vi "Host Train PID.vi"() -> ()   [LabVIEW 2018]
doc: "This example demonstrates the Traditional MeanShift algorithm to track an object in the image."
uses:
  <vilib>/userdefined/High Color/IMAQdx.ctl
  <vilib>/vision/driver/NI_Vision_Acquisition_Software.lvlib
panel:
  in  "?":T1="cam1"
  out "Control Sig":dbl(graph)
  out "Grn":bool
  out "Yel":bool
  out "Red":bool
  out "stop":bool
  out "global?":bool
  in  "Run":bool
  out "Theta":cluster{"Double":dbl, "Theta":dbl}(graph)
  out "Theta increasing?":bool
  in  "Stop":bool
  out "Image":T2(plugin-control)
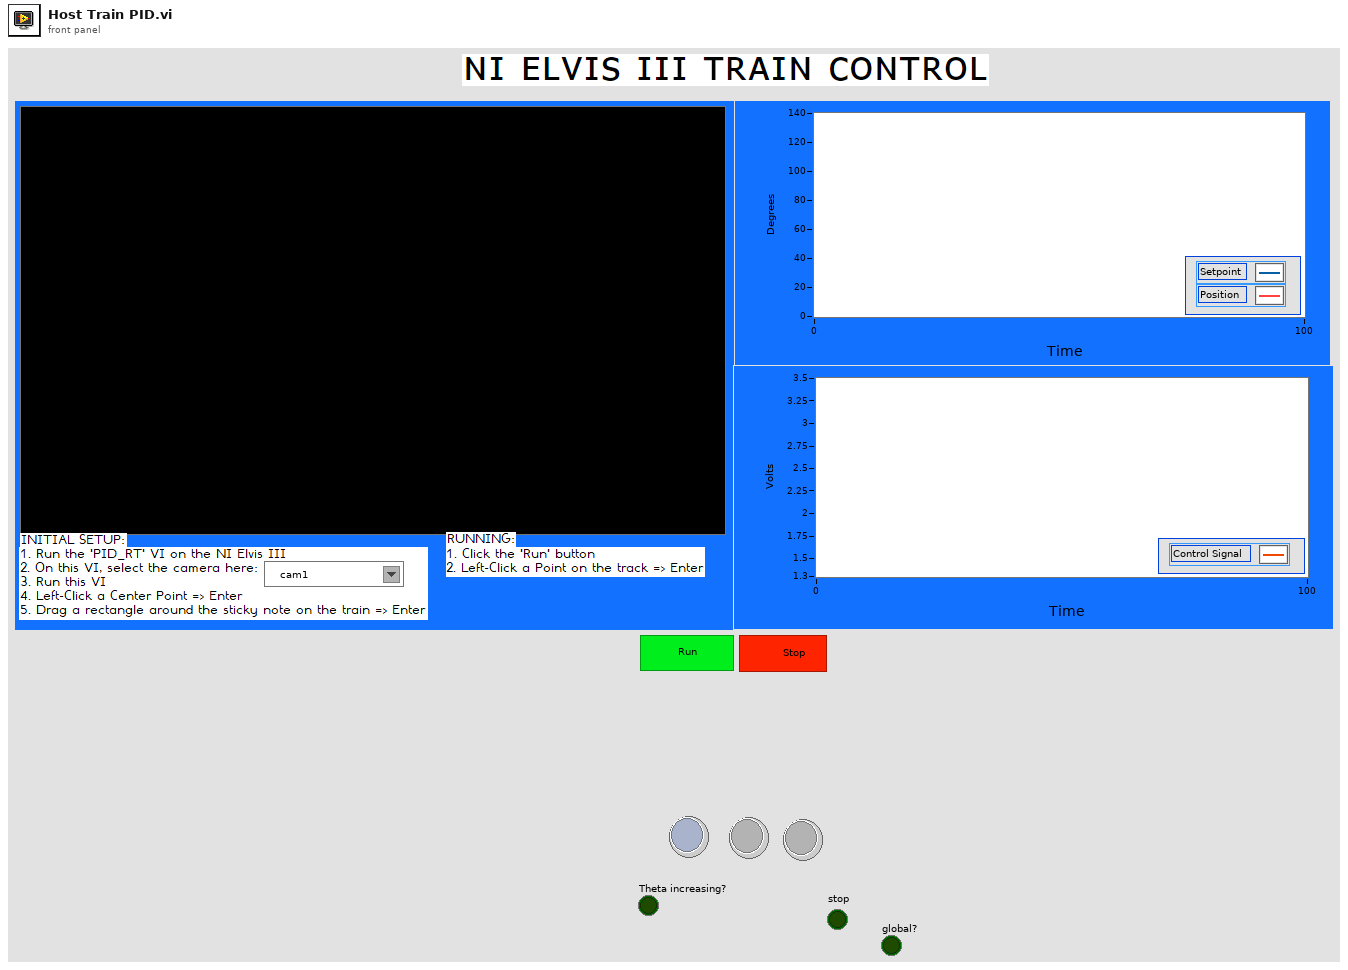
[diagram p1: front panel]
types:
  T1 = typedef "IMAQdx.ctl" = refnum<k21>
  T2 = typedef "IMAQ Image.ctl" = refnum<image>
  T3 = typedef "LVRectTypeDef.ctl" = cluster{"Left":i16, "Top":i16, "Right":i16, "Bottom":i16}
  T4 = typedef "IMAQ Object Tracking Session.ctl" = refnum<k20>
  T5 = typedef "IMAQ Point" = cluster{"X":sgl, "Y":sgl}
  T6 = cluster{"Label":string, "Score":i32, "Angle":dbl, "Location":cluster{"X":dbl, "Y":dbl}, "Bounding Box":cluster{"X":dbl, "Y":dbl}[], "Object Found?":bool}[]
  T7 = cluster{"Label":string, "Score":i32, "Angle":dbl, "Location":cluster{"X":dbl, "Y":dbl}, "Bounding Box":cluster{"X":dbl, "Y":dbl}[], "Object Found?":bool}
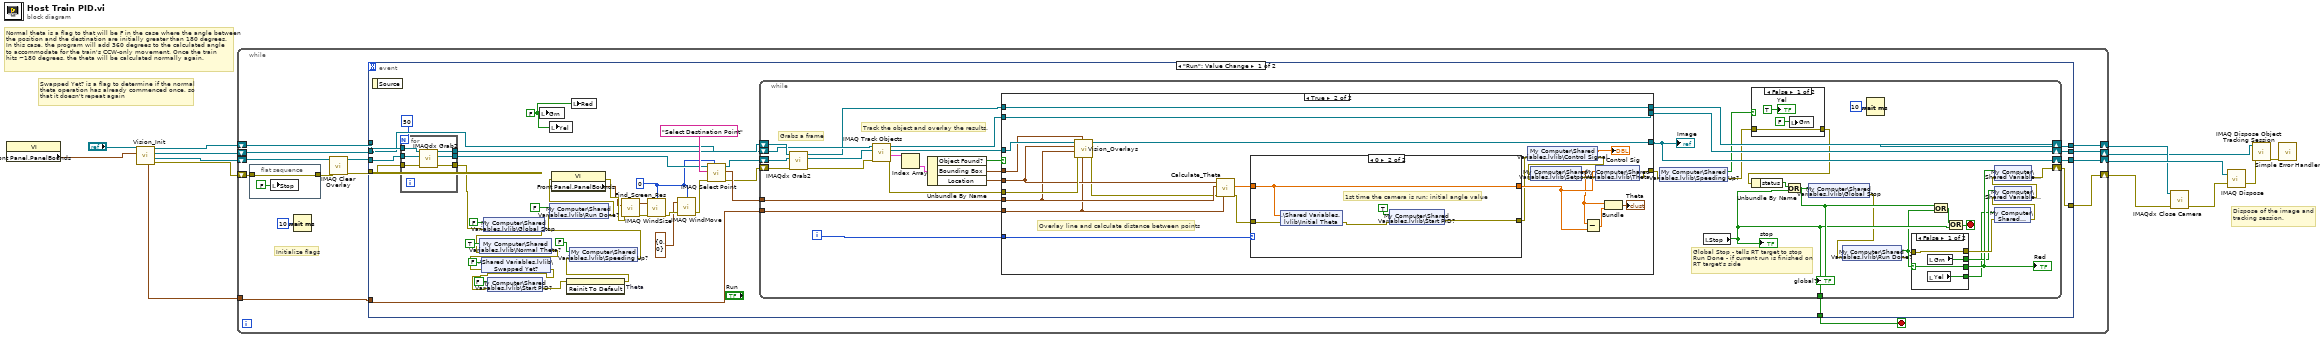
[diagram p0: block diagram]
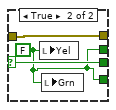
[diagram p2: hidden frame]
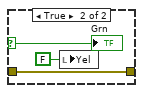
[diagram p3: hidden frame]
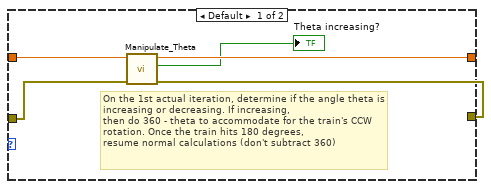
[diagram p5: hidden frame]
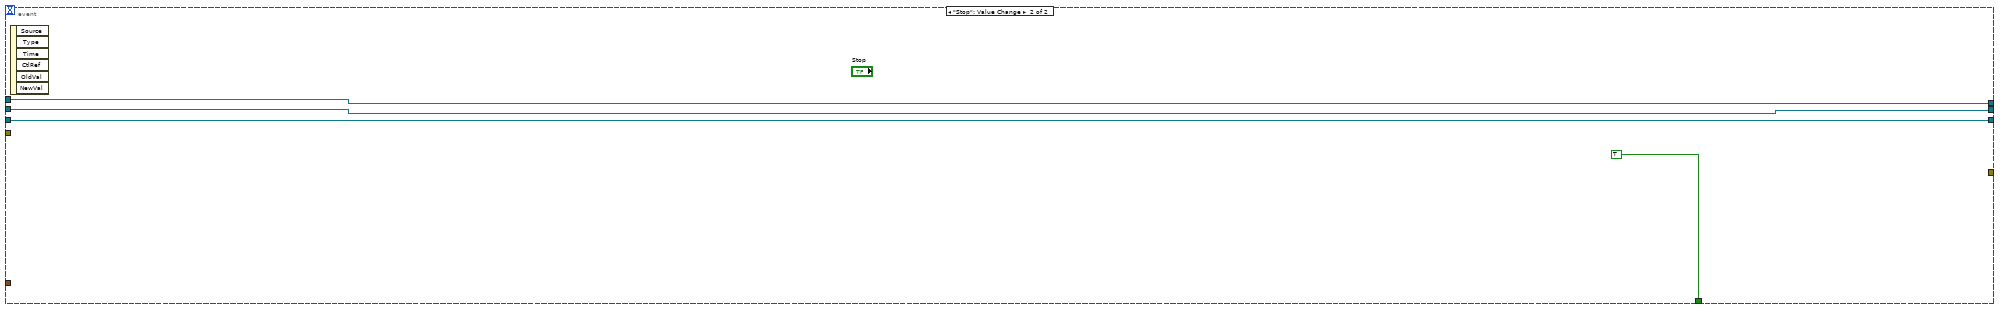
[diagram p6: hidden frame]
diagram:
  # "Swapped Yet? is a flag to determine if the normal\ntheta operation has already commenced once, so \nthat it doesn't repeat again"
  # "Normal theta is a flag to that will be F in the case where the angle between\nthe position and the destination are initially greater than 180 degrees. \nIn this case, the program will add 360 degrees to the calculated angle \nto accommodate for the train's CCW-only movement. Once the train\nhits ~180 degrees, the theta will be calculated normally again."
  # "Dispose of the image and tracking session."
  n1 = property class="VI"() -> ("Front Panel.PanelBounds"=w2:T3)  [unwired: 2 in, 2 out]
  n2 = call "Vision_Init.vi"("Front Panel.WinBounds"=w2, "Refnum in"="?") -> ("error out"=w7:errorcluster, "Image (duplicate)"=w8:T2, "Object Tracking Session Out"=w6:T4, "Refnum out"=w10:T1, "Center Point"=w5:T5)  [unwired: 5 in]
  n3 = while {
    tunnel: w5 -> [w26]
    shift-right: [w22] -> w3
    shift-left: w6 -> [w23]
    shift-right: [w28] -> w4
    shift-left: w10 -> [w24]
    shift-right: [w21] -> w9
    shift-left: w8 -> [w15]
    shift-right: [w27] -> w11
    shift-left: w7 -> [w20]
    stop <- w25 stop-if-true
    # "Initialize flags"
    n4 = flat-sequence {
      tunnel: w20 -> [w29]
      tunnel: [w29] -> w17
      frame #0 {
        n5 = local write "Stop"(FALSE ("Stop")) -> ()
      }
    }
    n6 = Wait (ms)(milliseconds to wait=u32 10) -> ()  [unwired: 1 out]
    n7 = call "IMAQ Clear Overlay"("error in (no error)"=w17, "Image"=w15) -> ("error out"=w16:errorcluster, "Image Out"=w18:T2)  [unwired: 8 in]
    n8 = event shown="[0] \"Run\": Value Change" {
      selector: _ -> [_ _]
      dyn-events: _ -> [_ _]
      timeout: _ -> [_ _]
      tunnel: w23 -> [w57 w168]
      tunnel: [w70 w169] -> w28
      tunnel: [w32 _] -> w27
      tunnel: [w69 w167] -> w21
      tunnel: w18 -> [w58 w167]
      tunnel: w26 -> [w68 _]
      tunnel: [w67 TRUE ("Stop")] -> w25
      tunnel: w24 -> [w62 w169]
      tunnel: [w63 w168] -> w22
      tunnel: w16 -> [w45 _]
      event "Run": Value Change {
        w31 = FALSE ("Grn")
        w39 = 0 ("Window Number")
        n9 = event-data() -> ()  [unwired: 1 in, 1 out]
        n10 = for {
          N: 50 -> [_]
          tunnel: w62 -> [w76]
          tunnel: [w75] -> w51
          tunnel: [w74] -> w60
          tunnel: [w73] -> w61
          tunnel: w58 -> [w72]
          tunnel: w45 -> [w71]
          n11 = call <vilib>:"IMAQdx Grab2.vi"("error in"=w71, "Image In"=w72, "Session In"=w76) -> ("error out"=w75:errorcluster, "Image Out"=w74:T2, "Session Out"=w73:T1)  [unwired: 5 in, 1 out]
        }
        n12 = shared-variable "My Computer\\Shared Variables.lvlib\\Global Stop"(FALSE ("Global Stop"), error in=w51) -> (error out=w50:errorcluster)
        n13 = shared-variable "My Computer\\Shared Variables.lvlib\\Normal Theta?"(TRUE ("Add 360?"), error in=w50) -> (error out=w49:errorcluster)
        n14 = shared-variable ".\\Shared Variables.lvlib\\Swapped Yet?"(FALSE ("Swapped Yet?"), error in=w49) -> (error out=w47:errorcluster)
        n15 = shared-variable "My Computer\\Shared Variables.lvlib\\Start PID?"(FALSE ("Start PID?"), error in=w47) -> (error out=w46:errorcluster)
        n16 = local write "Grn"(w31) -> ()
        n17 = local write "Yel"(w31) -> ()
        n18 = invoke on="Theta" class="WFChart (strict)" method="Reinit To Default"(error in=w46) -> (error out=w35:errorcluster)  [unwired: 2 in, 2 out]
        n19 = shared-variable "My Computer\\Shared Variables.lvlib\\Speeding Up?"(FALSE ("Speeding Up?"), error in=w35) -> (error out=w34:errorcluster)
        n20 = shared-variable "My Computer\\Shared Variables.lvlib\\Run Done?"(FALSE ("Run Done?"), error in=w34) -> (error out=w38:errorcluster)
        n21 = property class="VI"(error in=w38) -> (error out=w37:errorcluster, "Front Panel.PanelBounds"=w36:T3)  [unwired: 1 in, 1 out]
        n22 = local write "Red"(w31) -> ()
        n23 = call "Find_Screen_Res.vi"("error in (no error)"=w37, "Front Panel.WinBounds"=w36) -> ("error out"=w44:errorcluster, "Width & Height"=w43:cluster{"Width":i32, "Height":i32})  [unwired: 8 in]
        n24 = call "IMAQ WindSize"("error in (no error)"=w44, "Width & Height"=w43, "Window Number"=w39) -> ("error out"=w42:errorcluster)  [unwired: 3 in, 2 out]
        n25 = call "IMAQ WindMove"("Window Number (0...15)"=w39, "Coordinates (screen)"=cluster{"X Position":i32, "Y Position":i32} {"X Position"=0, "Y Position"=0}, "error in (no error)"=w42) -> ("error out"=w41:errorcluster)  [unwired: 2 in, 1 out]
        n26 = call "IMAQ Select Point"("Window Number (0...15)"=w39, "error in (no error)"=w41, "Prompt"="Select Destination Point", "Image In"=w60) -> ("error out"=w59:errorcluster, "Point"=w65:T5, "Image Out (duplicate)"=w64:T2)  [unwired: 4 in, 1 out]
        n27 = while {
          shift-right: [w80] -> w32
          shift-left: w59 -> [w117]
          shift-right: [w94] -> w70
          shift-left: w61 -> [w101]
          tunnel: w65 -> [w113]
          shift-right: [w93] -> w69
          shift-left: w64 -> [w114]
          tunnel: w68 -> [w112]
          tunnel: [w91] -> w67
          shift-right: [w96] -> w63
          shift-left: w57 -> [w100]
          i -> [w116]
          stop <- w110 stop-if-true
          # "Global Stop - tells RT target to stop\nRun Done - if current run is finished on\nRT target's side"
          # "Track the object and overlay the results."
          # "Grabs a frame"
          n28 = call <vilib>:"IMAQdx Grab2.vi"("error in"=w117, "Image In"=w114, "Session In"=w101) -> ("error out"=w102:errorcluster, "Image Out"=w92:T2, "Session Out"=w95:T1)  [unwired: 5 in, 1 out]
          n29 = call "IMAQ Track Objects"("error in (no error)"=w102, "Image"=w92, "Object Tracking Session In"=w100) -> ("error out"=w106:errorcluster, "Objects (pixel)"=w109:T6, "Image (duplicate)"=w108:T2, "Object Tracking Session Out"=w97:T4)  [unwired: 1 in, 4 out]
          n30 = Index Array(array=w109) -> (element=w105:T7)  [unwired: 1 in]
          n31 = Unbundle By Name(w105) -> ("Object Found?"=w104:bool, "Bounding Box"=w107:cluster{"X":dbl, "Y":dbl}[], "Location"=w103:cluster{"X":dbl, "Y":dbl})
          n32 = case shown="True" w104 {
            tunnel: w108 -> [w133 w156]
            tunnel: [w133 w138] -> w93
            tunnel: w107 -> [_ w154]
            tunnel: w106 -> [w134 w155]
            tunnel: [w134 w141] -> w90
            tunnel: w103 -> [_ w153]
            tunnel: w113 -> [_ w152]
            tunnel: w112 -> [_ w150]
            tunnel: w116 -> [_ w149]
            tunnel: w97 -> [w131 w144]
            tunnel: [w131 w144] -> w96
            tunnel: w95 -> [w132 w143]
            tunnel: [w132 w143] -> w94
            frame False {
            }
            frame True {
              # "Overlay line and calculate distance between points"
              n33 = call "Vision_Overlays.vi"("Center"=w150, "Bounding Box"=w154, "error in (no error)"=w155, "Destination"=w152, "Position"=w153, "Image in"=w156) -> ("error out"=w151:errorcluster, "Image out"=w138:T2)  [unwired: 4 in]
              n34 = call "Calculate_Theta.vi"("Center"=w150, "error in"=w151, "Destination"=w152, "Position"=w153) -> ("error out"=w148:errorcluster, "Theta"=w147:dbl)  [unwired: 6 in]
              n35 = case shown="0" w149 {
                tunnel: w147 -> [w161 w165]
                tunnel: w148 -> [w158 w166]
                tunnel: [w159 w162] -> w137
                tunnel: [w160 w165] -> w140
                frame Default {
                  # "On the 1st actual iteration, determine if the angle theta is increasing or decreasing. If increasing, \nthen do 360 - theta to accommodate for the train's CCW rotation. Once the train hits 180 degrees,\nresume normal calculations (don't subtract 360)"
                  n36 = call "Manipulate_Theta.vi"("error in (no error)"=w158, "Theta in"=w161) -> ("error out"=w159:errorcluster, "Boolean"=→"Theta increasing?":bool, "Theta out"=w160:dbl)  [unwired: 7 in]
                }
                frame 0 {
                  # "1st time the camera is run; initial angle value"
                  n37 = shared-variable ".\\Shared Variables.lvlib\\Initial Theta"(w165, error in=w166) -> (error out=w163:errorcluster)
                  n38 = shared-variable "My Computer\\Shared Variables.lvlib\\Start PID?"(TRUE ("Start PID?"), error in=w163) -> (error out=w162:errorcluster)
                }
              }
              n39 = shared-variable "My Computer\\Shared Variables.lvlib\\Control Signal"(error in=w137) -> (→"Control Sig":dbl, error out=w136:errorcluster)
              n40 = shared-variable "My Computer\\Shared Variables.lvlib\\Setpoint"(error in=w136) -> (w139:dbl, error out=w142:errorcluster)
              n41 = Subtract(x=w139, y=w140) -> (x-y=w145:dbl)
              n42 = shared-variable "My Computer\\Shared Variables.lvlib\\Theta"(w140, error in=w142) -> (error out=w141:errorcluster)
              n43 = Bundle("Double"=w139, w145) -> (→"Theta":cluster{"Double":dbl, dbl})  [unwired: 1 in]
            }
          }
          "Image" <- w93
          n44 = shared-variable "My Computer\\Shared Variables.lvlib\\Speeding Up?"(error in=w90) -> (w89:bool, error out=w87:errorcluster)
          n45 = local read "Stop"() -> (w91:bool)
          "stop" <- w91
          n46 = case shown="False" w89 {
            selector: w89 -> [_ w130]
            tunnel: w87 -> [w127 w129]
            tunnel: [w127 w129] -> w86
            frame False {
              n47 = local write "Grn"(FALSE ("Grn")) -> ()
              "Yel" <- TRUE ("Yel")
            }
            frame True {
              n48 = local write "Yel"(FALSE ("Yel")) -> ()
              "Grn" <- w130
            }
          }
          n49 = Unbundle By Name(w86) -> ("status"=w111:bool)
          n50 = Or(x=w111, y=w91) -> (x .or. y?=w99:bool)
          "global?" <- w99
          n51 = shared-variable "My Computer\\Shared Variables.lvlib\\Global Stop"(w99) -> (error out=w85:errorcluster)  [unwired: 1 in]
          n52 = shared-variable "My Computer\\Shared Variables.lvlib\\Run Done?"(error in=w85) -> (w88:bool, error out=w84:errorcluster)
          n53 = Wait (ms)(milliseconds to wait=u32 10) -> ()  [unwired: 1 out]
          n54 = case shown="False" w88 {
            selector: w88 -> [w120 w123]
            tunnel: w84 -> [w121 w124]
            tunnel: [w121 w124] -> w83
            tunnel: [w120 w123] -> w79
            tunnel: [w119 w122] -> w78
            tunnel: [w118 w122] -> w77
            frame False {
              n55 = local read "Grn"() -> (w119:bool)
              n56 = local read "Yel"() -> (w118:bool)
            }
            frame True {
              w122 = FALSE ("Yel")
              n57 = local write "Yel"(w122) -> ()
              n58 = local write "Grn"(w122) -> ()
            }
          }
          "Red" <- w79
          n59 = Or(x=w99, y=w88) -> (x .or. y?=w98:bool)
          n60 = Or(x=w98, y=w91) -> (x .or. y?=w110:bool)
          n61 = shared-variable "My Computer\\Shared Variables.lvlib\\Yel"(w77, error in=w83) -> (error out=w82:errorcluster)
          n62 = shared-variable "My Computer\\Shared Variables.lvlib\\Grn"(w78, error in=w82) -> (error out=w81:errorcluster)
          n63 = shared-variable "My Computer\\Shared Variables.lvlib\\Red"(w79, error in=w81) -> (error out=w80:errorcluster)
        }
      }
      event "Stop": Value Change {
        n64 = event-data() -> ()  [unwired: 1 in, 6 out]
      }
    }
  }
  n65 = call <vilib>:"IMAQdx Close Camera.vi"("error in"=w11, "Session In"=w4) -> ("error out"=w12:errorcluster)  [unwired: 9 in]
  n66 = call "IMAQ Dispose"("Image"=w9, "error in (no error)"=w12) -> ("error out"=w14:errorcluster)  [unwired: 1 in, 3 out]
  n67 = call "IMAQ Dispose Object Tracking Session"("error in (no error)"=w14, "Object Tracking Session"=w3) -> ("error out"=w13:errorcluster)  [unwired: 9 out]
  n68 = call <vilib>:"Simple Error Handler.vi"("error in (no error)"=w13) -> ()  [unwired: 1 in, 8 out]
